vi "CvrtCell2Data.vi"(8 "error in (no error)":errorcluster, 9 "ge_HdrNames":T1, 10 "Item Name":string, 11 "Resistance in":refnum<class "Resistance.lvclass">) -> (0 "error out":errorcluster, 3 "Resistance out":refnum<class "Resistance.lvclass">)   [LabVIEW 2012, in "Measurement Channels.lvlib" / "Resistance.lvclass"]
uses:
  Resistance.lvclass
  Common/Controls/HeaderNames.ctl
  Class Channel/Channel.lvclass
  SubVIs Table/Custom Ctls Table/ge_ColType.ctl
  Resistance.lvclass/Resistance.ctl
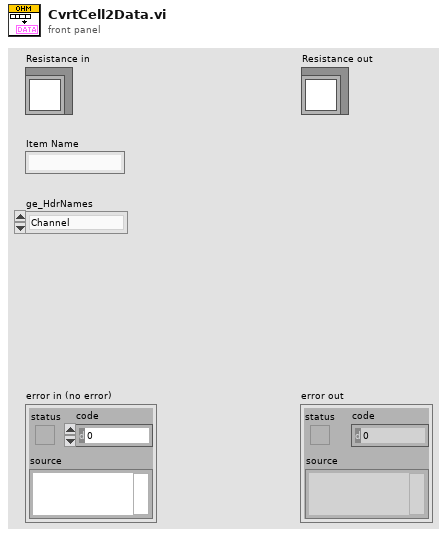
[diagram p1: front panel]
types:
  T1 = typedef "HeaderNames.ctl" = enum16{"Channel", "Device", "Spacer", "Description", "MB", "Range", "Terminal", "Coupling", "Thresh (V)", "Pulse/Rev", "Slope", "Min EU", "Min RPM", "mV/EU", "Iex", "Temp Units", "Type", "CJC Src", "CJC Val", "Ro", "Wire Cfg", "Strain Mode", "Vex", "Bridge Type", "GF", "Gauge Res", "Poisson", "Lead Res", "Init Strain", "GAF", "Scale", "Offset", "Unit (EU)", "dB?", "dB Ref", "Cal Mag", "Cal Units", "Max Temp", "Min Temp", "Max Strain", "Min Strain"}
  T2 = typedef "ge_ColType.ctl" = enum16{"Volts", "Amps", "Ohms", "TermCfg", "WireCfg", "Coup", "Slope", "Iex", "CalUnits", "ThrmUnits", "ThrmType", "CJCSrc", "BrdgType", "Strn Mode", "RTDType"}
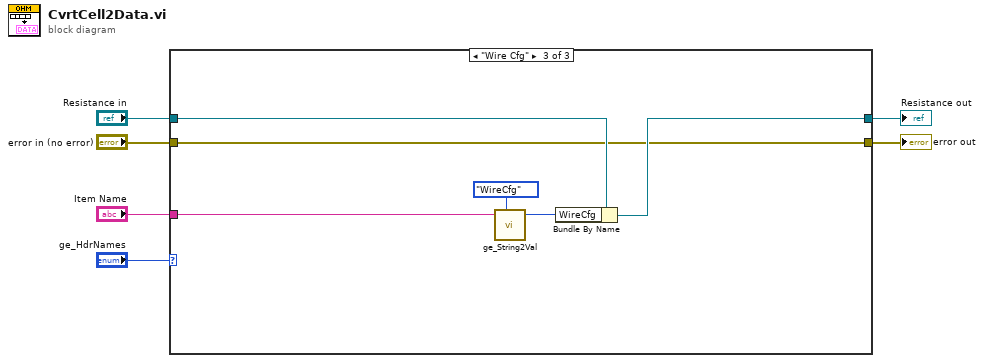
[diagram p0: block diagram]
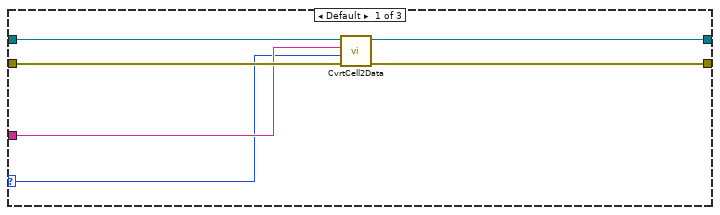
[diagram p2: hidden frame]
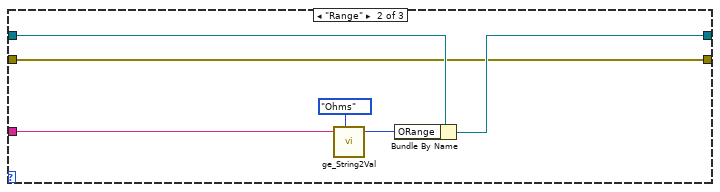
[diagram p3: hidden frame]
diagram:
  n1 = case shown="\"Wire Cfg\"" "ge_HdrNames" {
    selector: "ge_HdrNames" -> [w7 _ _]
    tunnel: "error in (no error)" -> [w12 w16 w22]
    tunnel: [w11 w16 w22] -> w5
    tunnel: [w10 w17 w23] -> w4
    tunnel: "Resistance in" -> [w9 w18 w24]
    tunnel: "Item Name" -> [w8 w13 w19]
    frame Default {
      n2 = call-parent "CvrtCell2Data.vi"("error in (no error)"=w12, "Header Names"=w7, "Item Name"=w8, "Channel in"=w9) -> ("error out"=w11:errorcluster, "Channel out"=w10:refnum<class "Resistance.lvclass">)  [unwired: 6 in]
    }
    frame "Range" {
      n3 = call "ge_String2Val.vi"("String"=w13, "ColType"=ge_ColType."Ohms") -> ("Value"=w14:u16)  [unwired: 4 in, 1 out]
      n4 = Bundle By Name(cluster=w18, "ORange"=w14) -> (w17:refnum<class "Resistance.lvclass">)
    }
    frame "Wire Cfg" {
      n5 = call "ge_String2Val.vi"("String"=w19, "ColType"=ge_ColType."WireCfg") -> ("Value"=w20:u16)  [unwired: 4 in, 1 out]
      n6 = Bundle By Name(cluster=w24, "WireCfg"=w20) -> (w23:refnum<class "Resistance.lvclass">)
    }
  }
  "error out" <- w5
  "Resistance out" <- w4
